vi "I16 To DBL.vi"(10 "Audio Data (1D I16)":i16[](array[numeric]), 11 "Audio Data (2D I16)":i16[][](array[numeric])) -> (2 "Audio Data (1D DBL)":dbl[](array[numeric]), 3 "Audio Data (2D DBL)":dbl[][](array[numeric]))   [LabVIEW 2019, in "Audio Processing.lvlib"]
doc: "Converts audio in I16 format (range -32768 to 32767) to DBL (range -1 to 1).\n\nWire 1D array for single channel audio, or 2D array for multi-channel audio."
uses:
  Audio Processing.lvlib
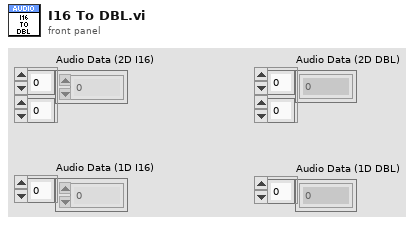
[diagram p1: front panel]
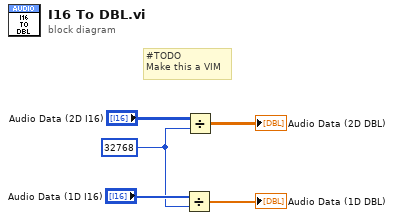
[diagram p0: block diagram]
diagram:
  w2 = 32768
  # "#TODO\nMake this a VIM"
  n1 = Divide(x="Audio Data (1D I16)", y=w2) -> (x/y=→"Audio Data (1D DBL)":dbl[])
  n2 = Divide(x="Audio Data (2D I16)", y=w2) -> (x/y=→"Audio Data (2D DBL)":dbl[][])
